vi "WPI_CameraIPCameraRead.vi"(0 "Refnum in":T1, 1 "Operation":enum16{"Read", "Reopen", "Close"}(ring), 2 "port":u16=80, 5 "address":string, 7 "cgi string":string, 9 "millisecs in":u32, 11 "error in (no error)":errorcluster, 12 "accum length in":i32, 13 "Authenticate":bool=TRUE) -> (4 "Refnum out":T1, 6 "length":i32, 8 "accum length out":i32, 10 "millisecs out":u32, 15 "error out":errorcluster)   [LabVIEW 2017]
uses:
  <vilib>/vision/Image Controls.llb/IMAQ Image.ctl
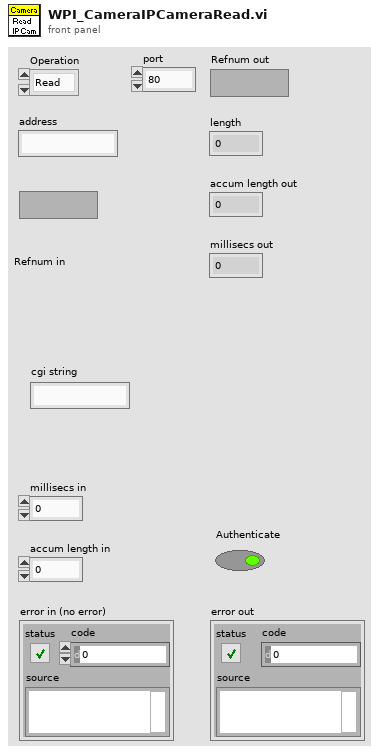
[diagram p1: front panel]
types:
  T1 = typedef "IMAQ Image.ctl" = refnum<image>
  T2 = enum16{"Standard", "Buffered", "CRLF", "Immediate"}
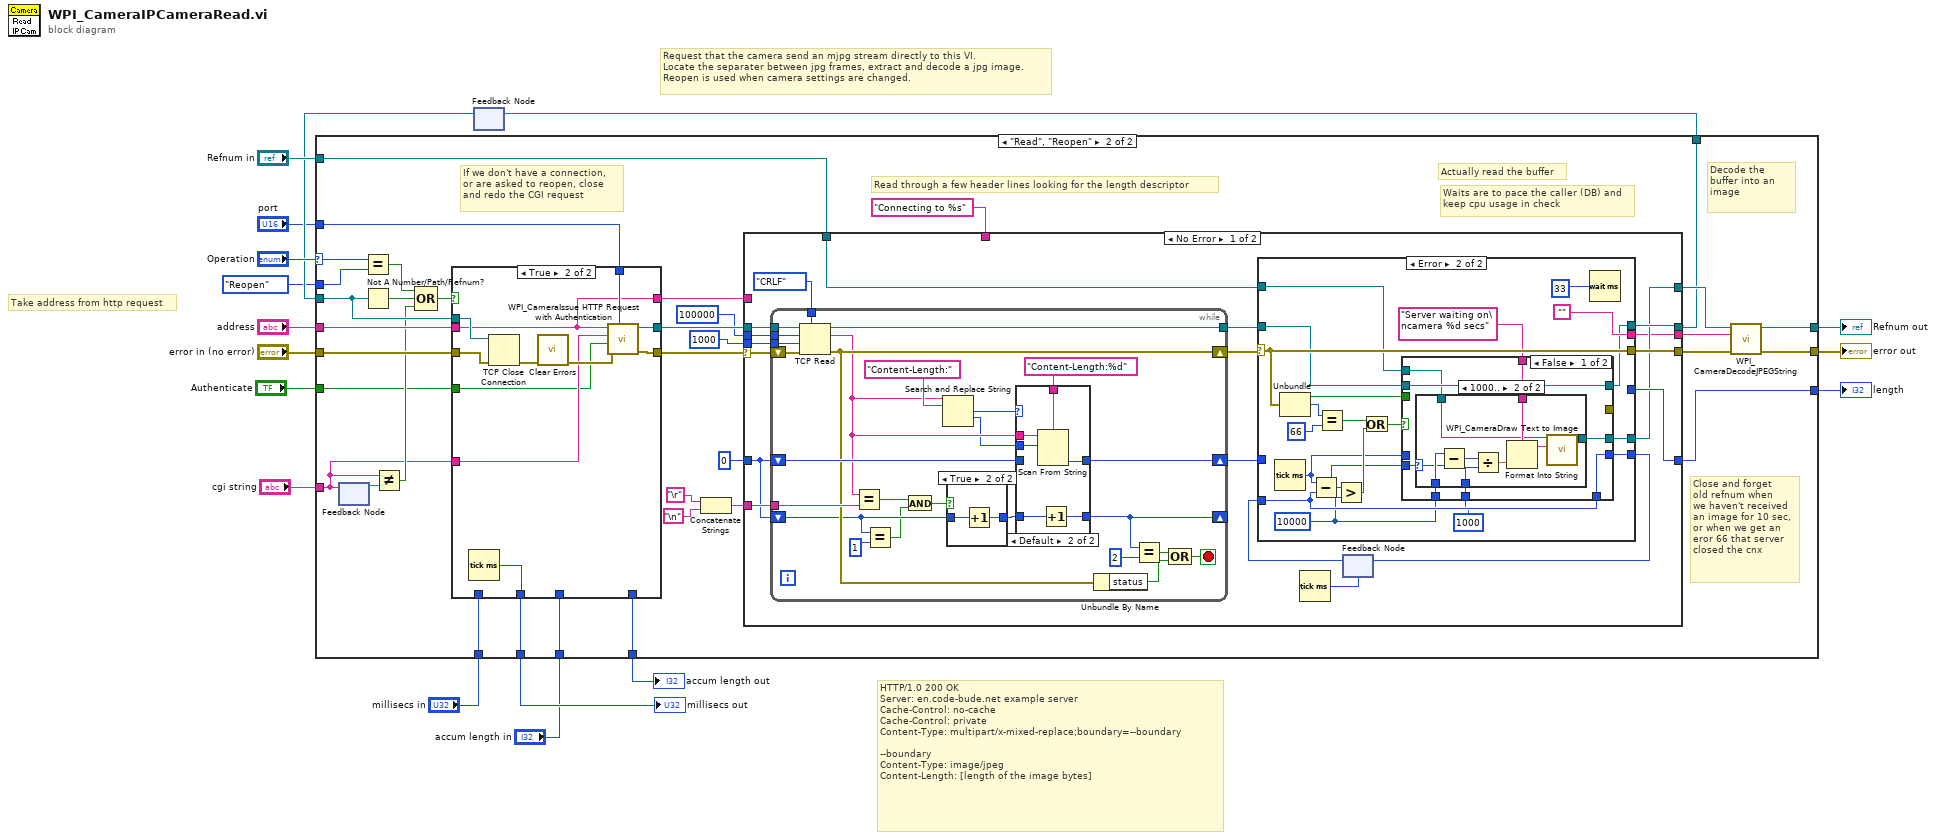
[diagram p0: block diagram]
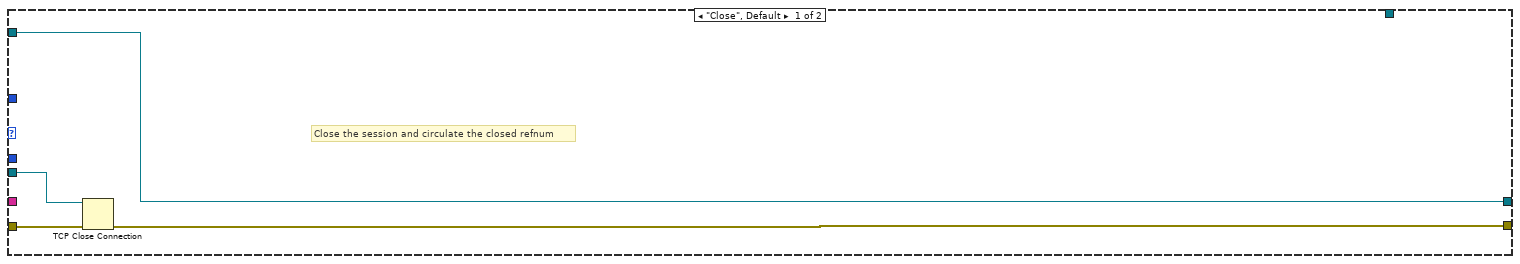
[diagram p2: hidden frame]
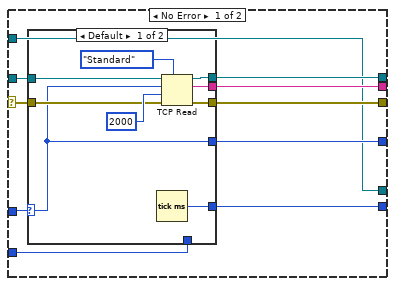
[diagram p4: hidden frame]
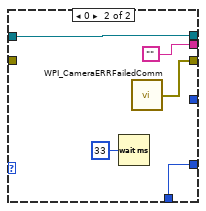
[diagram p5: hidden frame]
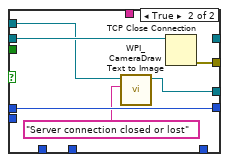
[diagram p7: hidden frame]
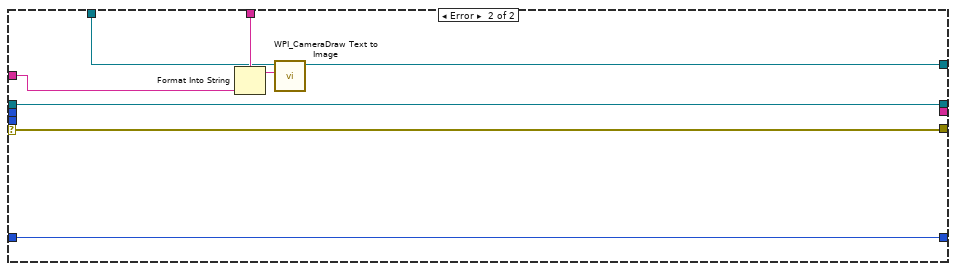
[diagram p10: hidden frame]
diagram:
  # "HTTP/1.0 200 OK\nServer: en.code-bude.net example server\nCache-Control: no-cache\nCache-Control: private\nContent-Type: multipart/x-mixed-replace;boundary=--boundary\n \n--boundary\nContent-Type: image/jpeg\nContent-Length: [length of the image bytes]"
  # "Take address from http request"
  # "Request that the camera send an mjpg stream directly to this VI.\nLocate the separater between jpg frames, extract and decode a jpg image.\nReopen is used when camera settings are changed."
  n1 = feedback #1() -> (w10:refnum<k5>)  [unwired: 1 out]
  n2 = case shown="\"Read\", \"Reopen\"" "Operation" {
    selector: "Operation" -> [_ w44]
    tunnel: "error in (no error)" -> [w20 w50]
    tunnel: "address" -> [_ w49]
    tunnel: [_ w25] -> w7
    tunnel: "cgi string" -> [_ w32]
    tunnel: [w18 w47] -> w8
    tunnel: [w19 w46] -> w9
    tunnel: w10 -> [w21 w45]
    tunnel: "Refnum in" -> [w18 w28]
    tunnel: [_ w24] -> w13
    tunnel: "accum length in" -> [_ w43]
    tunnel: [_ w42] -> w15
    tunnel: "millisecs in" -> [_ w41]
    tunnel: [_ w40] -> w17
    tunnel: enum16{"Read", "Reopen", "Close"}."Reopen" ("Operation") -> [_ w34]
    tunnel: "port" -> [_ w33]
    tunnel: "Authenticate" -> [_ w30]
    frame "Close", Default {
      # "Close the session and circulate the closed refnum"
      n3 = TCP Close Connection(connection ID=w21, error in (no error)=w20) -> (error out=w19:errorcluster)  [unwired: 2 out]
    }
    frame "Read", "Reopen" {
      # "Waits are to pace the caller (DB) and\nkeep cpu usage in check"
      # "Close and forget\nold refnum when\nwe haven't received\nan image for 10 sec,\nor when we get an\neror 66 that server\nclosed the cnx"
      # "Decode the buffer into an image"
      # "Actually read the buffer"
      # "Read through a few header lines looking for the length descriptor"
      # "If we don't have a connection,\nor are asked to reopen, close\nand redo the CGI request"
      n4 = feedback #2() -> (w39:string)  [unwired: 1 out]
      n5 = feedback-in #2(w32) -> ()
      n6 = Equal?(x=w44, y=w34) -> (x = y?=w38:bool)
      n7 = Not A Number/Path/Refnum?(number/path/refnum=w45) -> (NaN/Path/Refnum?=w37:bool)
      n8 = Not Equal?(x=w32, y=w39) -> (x != y?=w35:bool)
      n9 = Compound Arithmetic op=OR(w38, w37, w35) -> (w36:bool)
      n10 = case shown="True" w36 {
        tunnel: [w60 w71] -> w53
        tunnel: [w61 w72] -> w52
        tunnel: w50 -> [w60 w69]
        tunnel: w49 -> [w57 w62]
        tunnel: w45 -> [w61 w70]
        tunnel: w43 -> [w59 _]
        tunnel: [w59 _] -> w42
        tunnel: w41 -> [w58 _]
        tunnel: [w58 w66] -> w40
        tunnel: w33 -> [_ w65]
        tunnel: w32 -> [_ w64]
        tunnel: w30 -> [_ w63]
        tunnel: [w57 w62] -> w27
        frame False {
        }
        frame True {
          n11 = Tick Count (ms)() -> (millisecond timer value=w66:u32)
          n12 = TCP Close Connection(connection ID=w70, error in (no error)=w69) -> (error out=w68:errorcluster)  [unwired: 2 out]
          n13 = call <vilib>:"Clear Errors.vi"("error in (no error)"=w68) -> ("error out"=w67:errorcluster)  [unwired: 1 in, 5 out]
          n14 = call <vilib>:"WPI_CameraIssue HTTP Request with Authentication.vi"("port"=w65, "error in (no error)"=w67, "Authenticate"=w63, "Request"=w64, "address"=w62) -> ("error out"=w71:errorcluster, "connection ID (dup)"=w72:refnum<k5>)  [unwired: 5 out]
        }
      }
      n15 = Concatenate Strings("\r", "\n") -> (w54:string)
      n16 = case shown="No Error" w53 {
        selector: w53 -> [w87 w203]
        tunnel: [w76 w203] -> w23
        tunnel: [w77 w202] -> w24
        tunnel: [w75 w204] -> w25
        tunnel: w54 -> [w91 _]
        tunnel: w52 -> [w89 w204]
        tunnel: 1000 ("bytes to read") -> [w88 _]
        tunnel: 0 -> [w86 w202]
        tunnel: 100000 ("bytes to read") -> [w85 _]
        tunnel: [w74 w200] -> w26
        tunnel: "Connecting to %s" ("regular expression") -> [_ w199]
        tunnel: w28 -> [w81 w198]
        tunnel: w27 -> [_ w197]
        tunnel: [w73 _] -> w22
        frame No Error {
          n17 = while {
            tunnel: w89 -> [w185]
            tunnel: [w184] -> w80
            shift-right: [w183] -> w78
            shift-left: w86 -> [w182]
            shift-right: [w165] -> _
            shift-left: w86 -> [w163]
            tunnel: w91 -> [w180]
            tunnel: w88 -> [w170]
            tunnel: T2."CRLF" ("mode (standard)") -> [w179]
            shift-right: [w177] -> w79
            shift-left: w87 -> [w178]
            tunnel: w85 -> [w168]
            stop <- w176 stop-if-true
            n18 = TCP Read(connection ID=w185, bytes to read=w168, error in (no error)=w178, 7:w179, 9:w170) -> (connection ID out=w184:refnum<k5>, data out=w171:string, error out=w177:errorcluster)
            n19 = Equal?(x=w171, y=w180) -> (x = y?=w161:bool)
            n20 = Equal?(x=w163, y=1) -> (x = y?=w162:bool)
            n21 = And(x=w161, y=w162) -> (x .and. y?=w160:bool)
            n22 = Search and Replace String(input string=w171, search string="Content-Length:" ("regular expression")) -> (number of replacements=w175:i32, offset past replacement=w169:i32)  [unwired: 1 in, 7 out]
            n23 = case shown="True" w160 {
              tunnel: w163 -> [w186 w188]
              tunnel: [w186 w187] -> w166
              frame False {
              }
              frame True {
                n24 = Increment(x=w188) -> (x+1=w187:i32)
              }
            }
            n25 = case shown="Default" w175 {
              tunnel: [w190 w196] -> w183
              tunnel: w182 -> [w190 _]
              tunnel: w171 -> [_ w195]
              tunnel: w169 -> [_ w194]
              tunnel: "Content-Length:%d" ("regular expression") -> [_ w193]
              tunnel: w166 -> [w189 w192]
              tunnel: [w189 w191] -> w165
              frame 0 {
              }
              frame Default {
                n26 = Scan From String(format string=w193, input string=w195, initial scan location=w194) -> (output 1=w196:i32)  [unwired: 1 in, 4 out]
                n27 = Increment(x=w192) -> (x+1=w191:i32)
              }
            }
            n28 = Unbundle By Name(w177) -> ("status"=w172:bool)
            n29 = Equal?(x=w165, y=2) -> (x = y?=w173:bool)
            n30 = Compound Arithmetic op=OR(w173, w172) -> (w176:bool)
          }
          n31 = Tick Count (ms)() -> (millisecond timer value=w82:u32)
          n32 = feedback #3(w82) -> (w83:u32)
          n33 = case shown="Error" w79 {
            selector: w79 -> [w97 w134]
            tunnel: [w101 w134] -> w76
            tunnel: [w100 ""] -> w73
            tunnel: [w99 w131] -> w75
            tunnel: w78 -> [w96 _]
            tunnel: w80 -> [w98 w132]
            tunnel: [w95 w125] -> w84
            tunnel: w83 -> [w94 w123]
            tunnel: [w93 _] -> w77
            tunnel: [w92 w117] -> w74
            tunnel: w81 -> [w92 w116]
            frame No Error {
              n34 = case shown="Default" w96 {
                selector: w96 -> [w102 _]
                tunnel: w98 -> [w110 w114]
                tunnel: [w109 w113] -> w101
                tunnel: [w106 ""] -> w100
                tunnel: [w105 w114] -> w99
                tunnel: w97 -> [w104 _]
                tunnel: [w103 w111] -> w95
                tunnel: w94 -> [_ w111]
                tunnel: [w102 _] -> w93
                frame Default {
                  n35 = Tick Count (ms)() -> (millisecond timer value=w103:u32)
                  n36 = TCP Read(connection ID=w110, bytes to read=w102, error in (no error)=w104, 7:T2."Standard" ("mode (standard)"), 9:2000 ("timeout ms (25000)")) -> (connection ID out=w105:refnum<k5>, data out=w106:string, error out=w109:errorcluster)
                }
                frame 0 {
                  n37 = Wait (ms)(milliseconds to wait=u32 33) -> ()  [unwired: 1 out]
                  n38 = call <vilib>:"WPI_CameraERRFailedComm.vi"() -> ("error out"=w113:errorcluster)
                }
              }
            }
            frame Error {
              w120 = u32 10000 ("milliseconds to wait")
              n39 = Tick Count (ms)() -> (millisecond timer value=w124:u32)
              n40 = Unbundle(w134) -> ("status"=w133:bool, "code"=w129:i32)  [unwired: 1 out]
              n41 = Subtract(x=w124, y=w123) -> (x-y=w121:u32)
              n42 = Equal?(x=w129, y=u32 66 ("milliseconds to wait")) -> (x = y?=w128:bool)
              n43 = Greater?(x=w121, y=w120) -> (0:w126:bool)
              n44 = Or(x=w128, y=w126) -> (x .or. y?=w127:bool)
              n45 = case shown="False" w127 {
                tunnel: w133 -> [_ _]
                tunnel: w132 -> [w143 w159]
                tunnel: [w143 _] -> w131
                tunnel: [w142 w158] -> w125
                tunnel: w124 -> [_ w158]
                tunnel: w123 -> [w142 _]
                tunnel: [_ w157] -> _
                tunnel: w121 -> [w141 _]
                tunnel: w120 -> [w140 _]
                tunnel: u32 1000 ("milliseconds to wait") -> [w139 _]
                tunnel: "Server waiting on\ncamera %d secs" ("regular expression") -> [w138 _]
                tunnel: [w137 w156] -> w117
                tunnel: w116 -> [w136 w155]
                frame False {
                  n46 = case shown="1000.." w141 {
                    selector: w141 -> [_ w152]
                    tunnel: w140 -> [_ w153]
                    tunnel: w139 -> [_ w150]
                    tunnel: w138 -> [_ w148]
                    tunnel: [w144 w146] -> w137
                    tunnel: w136 -> [w144 w145]
                    frame 0, Default {
                    }
                    frame 1000.. {
                      n47 = Subtract(x=w153, y=w152) -> (x-y=w151:u32)
                      n48 = Divide(x=w151, y=w150) -> (x/y=w149:dbl)
                      n49 = Format Into String(format string=w148, w149) -> (resulting string=w147:string)  [unwired: 2 in, 1 out]
                      n50 = call <vilib>:"WPI_CameraDraw Text to Image.vi"("Text"=w147, "Refnum in"=w145) -> ("Refnum out"=w146:T1)  [unwired: 9 in]
                    }
                  }
                }
                frame True {
                  n51 = call <vilib>:"WPI_CameraDraw Text to Image.vi"("Text"="Server connection closed or lost" ("regular expression"), "Refnum in"=w155) -> ("Refnum out"=w156:T1)  [unwired: 9 in]
                  n52 = TCP Close Connection(connection ID=w159) -> (error out=w157:errorcluster)  [unwired: 1 in, 2 out]
                }
              }
              n53 = Wait (ms)(milliseconds to wait=u32 33) -> ()  [unwired: 1 out]
            }
          }
          n54 = feedback-in #3(w84) -> ()
        }
        frame Error {
          n55 = Format Into String(format string=w199, w197) -> (resulting string=w201:string)  [unwired: 2 in, 1 out]
          n56 = call <vilib>:"WPI_CameraDraw Text to Image.vi"("Text"=w201, "Refnum in"=w198) -> ("Refnum out"=w200:T1)  [unwired: 9 in]
        }
      }
      n57 = call <vilib>:"WPI_CameraDecodeJPEGString.vi"("error in"=w23, "Compressed Image"=w22, "Image In"=w26) -> ("error out"=w46:errorcluster, "Image Out"=w47:T1)  [unwired: 3 out]
    }
  }
  "millisecs out" <- w17
  "accum length out" <- w15
  "length" <- w13
  "error out" <- w9
  "Refnum out" <- w8
  n58 = feedback-in #1(w7) -> ()
